vi "_Add Part.vi"(8 "error in":errorcluster, 10 "PartType":i32(ring) items=["Worksheet", "SharedString"], 11 "SpreadsheetDocument in":refnum<k24>) -> (0 "error out":errorcluster, 2 "OpenXmlPart":refnum<k24>, 3 "SpreadsheetDocument out":refnum<k24>)   [LabVIEW 2021, in "Open Xml.lvlib"]
uses:
  Open Xml.lvlib
  D:/git/Open-Xml-LabVIEW/dll/OpenXmlGenericsWrapper.dll
  dll/OpenXmlGenericsWrapper.dll
  D:/git/Open-Xml-LabVIEW/dll/DocumentFormat.OpenXml.dll
  dll/DocumentFormat.OpenXml.dll
  D:/git/Open-Xml-LabVIEW/dll/DocumentFormat.OpenXml.Framework.dll
  dll/DocumentFormat.OpenXml.Framework.dll
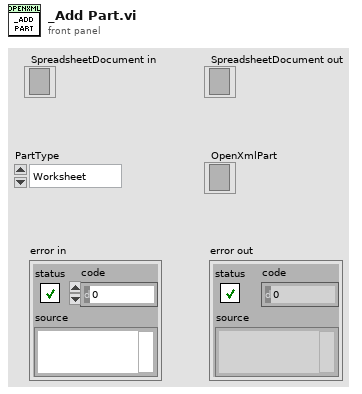
[diagram p1: front panel]
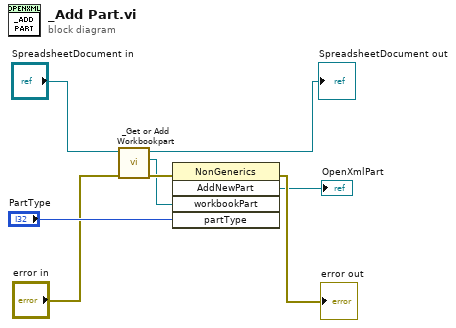
[diagram p0: block diagram]
diagram:
  n1 = call "_Get or Add Workbookpart.vi"("error in"="error in", "SpreadsheetDocument"="SpreadsheetDocument in") -> ("error out"=w6:errorcluster, "WorkbookPart"=w4:refnum<k24>, "SpreadsheetDocument out"=→"SpreadsheetDocument out":refnum<k24>)  [unwired: 7 in]
  n2 = invoke class="NonGenerics" method="AddNewPart"(error in=w6, "workbookPart"=w4, "partType"="PartType") -> (error out=→"error out":errorcluster, "AddNewPart"=→"OpenXmlPart":refnum<k24>)  [unwired: 2 in, 3 out]
